vi "meth.ExecFromFile.vi"(0 "class.GLue in":refnum<class "class.GLue.lvclass">, 2 "Path":path, 5 "Argument":variant, 11 "error in (no error)":errorcluster, 13 "ms timeout (-1)":i32=-1) -> (4 "class.GLue out":refnum<class "class.GLue.lvclass">, 6 "Return":variant, 15 "error out":errorcluster)   [LabVIEW 2014, in "GLue.lvlib" / "class.GLue.lvclass"]
uses:
  class.GLue.lvclass
  class.GLue.lvclass/class.GLue.ctl
  <vilib>/Utility/semaphor.llb/Acquire Semaphore.vi
  meth.RunChunk.vi
  <vilib>/Utility/semaphor.llb/Release Semaphore.vi
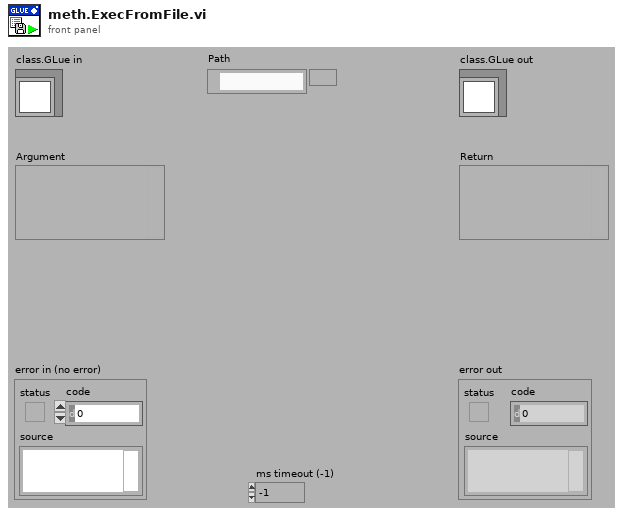
[diagram p1: front panel]
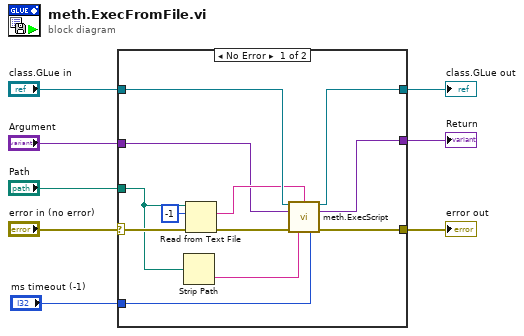
[diagram p0: block diagram]
diagram:
  n1 = case shown="No Error" "error in (no error)" {
    selector: "error in (no error)" -> [w16 w22]
    tunnel: [w20 w22] -> w7
    tunnel: [w19 w21] -> w5
    tunnel: "class.GLue in" -> [w18 w21]
    tunnel: "ms timeout (-1)" -> [w11 _]
    tunnel: "Argument" -> [w12 _]
    tunnel: [w17 _] -> w2
    tunnel: "Path" -> [w10 _]
    frame No Error {
      n2 = Strip Path(path=w10) -> (name=w9:string)  [unwired: 1 out]
      n3 = Read from Text File(file (use dialog)=w10, count=-1, error in=w16) -> (text=w13:string, error out=w15:errorcluster)  [unwired: 1 in, 2 out]
      n4 = call "meth.ExecScript.vi"("GLue in"=w18, "Script"=w13, "Argument"=w12, "error in"=w15, "Name"=w9, "ms timeout (-1)"=w11) -> ("GLue out"=w19:refnum<class "class.GLue.lvclass">, "Return"=w17:variant, "error out"=w20:errorcluster)  [unwired: 7 in]
    }
    frame Error {
    }
  }
  "error out" <- w7
  "class.GLue out" <- w5
  "Return" <- w2
